vi "Create Wheel Angular Velocity Row.vi"(8 "error in (no error)":errorcluster, 10 "steering angle (rad)":dbl, 11 "omni wheel in":refnum<class "NI_Robotics_Omnidirectional Wheel.lvclass">) -> (0 "error out":errorcluster, 2 "wheel angular velocity row":dbl[](array[numeric]), 3 "omni wheel out":refnum<class "NI_Robotics_Omnidirectional Wheel.lvclass">)   [LabVIEW 2017, in "NI_Robotics_Omnidirectional Wheel.lvclass"]
uses:
  <vilib>/robotics/Steering/Omnidirectional Wheel/NI_Robotics_Omnidirectional Wheel.lvclass
  c:/Program Files (x86)/National Instruments/LabVIEW 2017/vi.lib/robotics/Steering/Wheel/NI_Robotics_Wheel.lvclass
  <vilib>/robotics/Steering/Wheel/NI_Robotics_Wheel.lvclass/NI_Robotics_Wheel.ctl
  <vilib>/robotics/Steering/Wheel/NI_Robotics_Wheel.lvclass
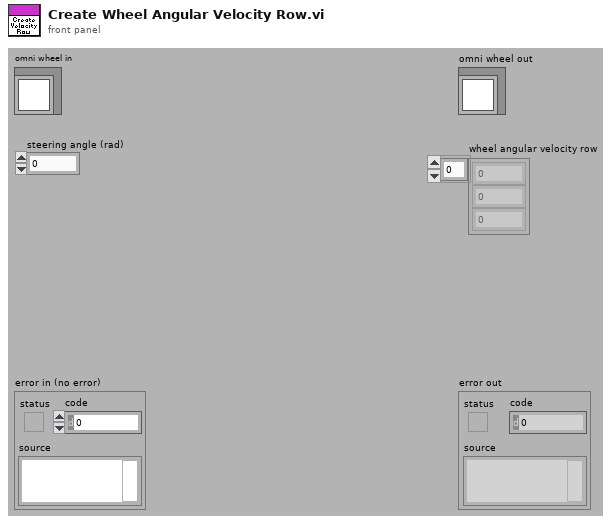
[diagram p1: front panel]
types:
  T1 = typedef "NI_Matrix.lvlib/RealMatrix.ctl" = dbl[][]
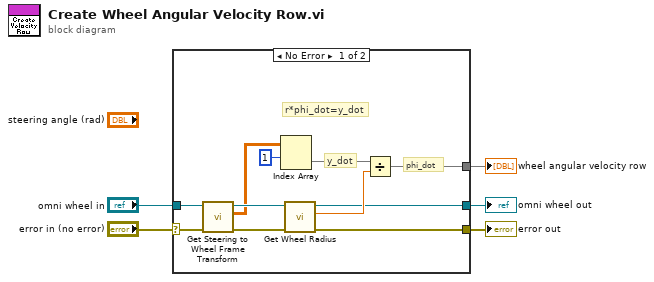
[diagram p0: block diagram]
diagram:
  n1 = case shown="No Error" "error in (no error)" {
    selector: "error in (no error)" -> [w8 w17]
    tunnel: "omni wheel in" -> [w10 w18]
    tunnel: [w13 w18] -> w3
    tunnel: [w12 _] -> w2
    tunnel: [w11 w17] -> w1
    frame No Error {
      # "phi_dot"
      # "r*phi_dot=y_dot"
      # "y_dot"
      n2 = call <vilib>:"Get Steering to Wheel Frame Transform.vi"("error in (no error)"=w8, "wheel in"=w10) -> ("error out"=w7:errorcluster, "steering to wheel frame transform"=w6:T1, "wheel out"=w9:refnum<class "NI_Robotics_Omnidirectional Wheel.lvclass">)  [unwired: 7 in]
      n3 = Index Array(array=w6, index (row)=1) -> (element=w15:dbl[])  [unwired: 1 in]
      n4 = call <vilib>:"Get Wheel Radius.vi"("error in (no error)"=w7, "wheel in"=w9) -> ("error out"=w11:errorcluster, "wheel radius"=w14:dbl, "wheel out"=w13:refnum<class "NI_Robotics_Omnidirectional Wheel.lvclass">)  [unwired: 7 in]
      n5 = Divide(x=w15, y=w14) -> (x/y=w12:dbl[])
    }
    frame Error {
    }
  }
  "error out" <- w1
  "omni wheel out" <- w3
  "wheel angular velocity row" <- w2
